vi "2810A Disconnect.vi"(8 "error in (no error)":errorcluster, 9 "Numeric":i32, 10 "Array":string[](array[string]), 11 "IVI Refnum in":refnum<k15>) -> (0 "error out":errorcluster, 3 "IVI Refnum out":refnum<k15>)   [LabVIEW 2019, in "SupportVIs.lvlib"]
uses:
  <instrlib>/niSwitch/niSwitch.llb/niSwitch Disconnect Channels (Multiple).vi
  SupportVIs.lvlib
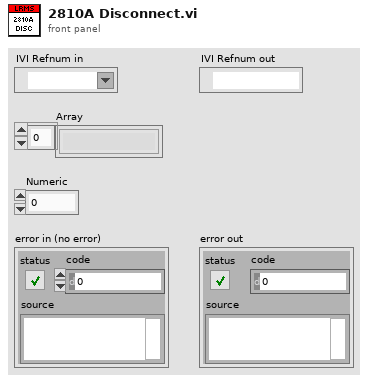
[diagram p1: front panel]
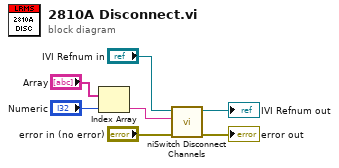
[diagram p0: block diagram]
diagram:
  n1 = Index Array(array="Array", index="Numeric") -> (element=w2:string)
  n2 = call-poly <instrlib>:"niSwitch Disconnect Channels.vi"("error in (no error)"="error in (no error)", "disconnection list"=w2, "instrument handle"="IVI Refnum in") -> ("error out"=→"error out":errorcluster, "instrument handle out"=→"IVI Refnum out":refnum<k15>)  [unwired: 7 in]
